vi "Call Steps.vi"(8 "error in (no error)":errorcluster, 11 "Cluster":T1={"Tite"="", "Base path"=path "", "Table"=[], "Stations"=[], "Shield Array"=[], "UPHs"=[], "VISA"={"VISA"="", "baud rate"=9600, "data bits"=8, "parity"=enum."None", "stop bits"=10, "flow control"=0}, "Path"={"roof"=path "", "Config"=path "", "Png"=path ""}, "Ctr"={"DB Dispaly"=refnum, "Error Table"=refnum, "Display"=refnum, "Login"=refnum, "Exit"=refnum, "FTT_Submit"=refnum}, "Login"={"User"="", "Grade"=""}, "information"={"cause"="", "Type"=enum."Inform", "code"=0, "Suroce"="", "Status"=FALSE}, "Local DB"={"Connstr"="", "Database"={"Constr"={"Driver"="", "Server"="", "User"="", "Pwd"="", "Database"=""}, "conn ref"=refnum, "State"=FALSE}}, "Remote DB"={"Connstr"="", "Database"={"Constr"={"Driver"="", "Server"="", "User"="", "Pwd"="", "Database"=""}, "conn ref"=refnum, "State"=FALSE}}, "FTT TV"="", "ExchangeTime"=0, "NVH"="", "EOL Path"=path ""} {"VISA"."flow control" items=["None", "XON/XOFF", "RTS/CTS", "XON/XOFF & RTS/CTS", "DTR/DSR", "XON/XOFF & DTR/DSR"]; "VISA"."stop bits" items=["1.0"=10, "1.5"=15, "2.0"=20]}) -> (0 "error out":errorcluster)   [LabVIEW 2014]
uses:
  Type'def/UPH Config.ctl
  VISA/Ctr/VISA Ctr.ctl
  Type'def/Main Ctr Ref.ctl
  Type'def/User Login.ctl
  Database/Ctr/Constr.ctl
  <vilib>/addons/database/Connection.llb/Conn ObjectReference.ctl
  <vilib>/addons/database/NI_Database_API.lvlib
  Database/Ctr/Conneect State.ctl
  Type'def/MainCtr.ctl
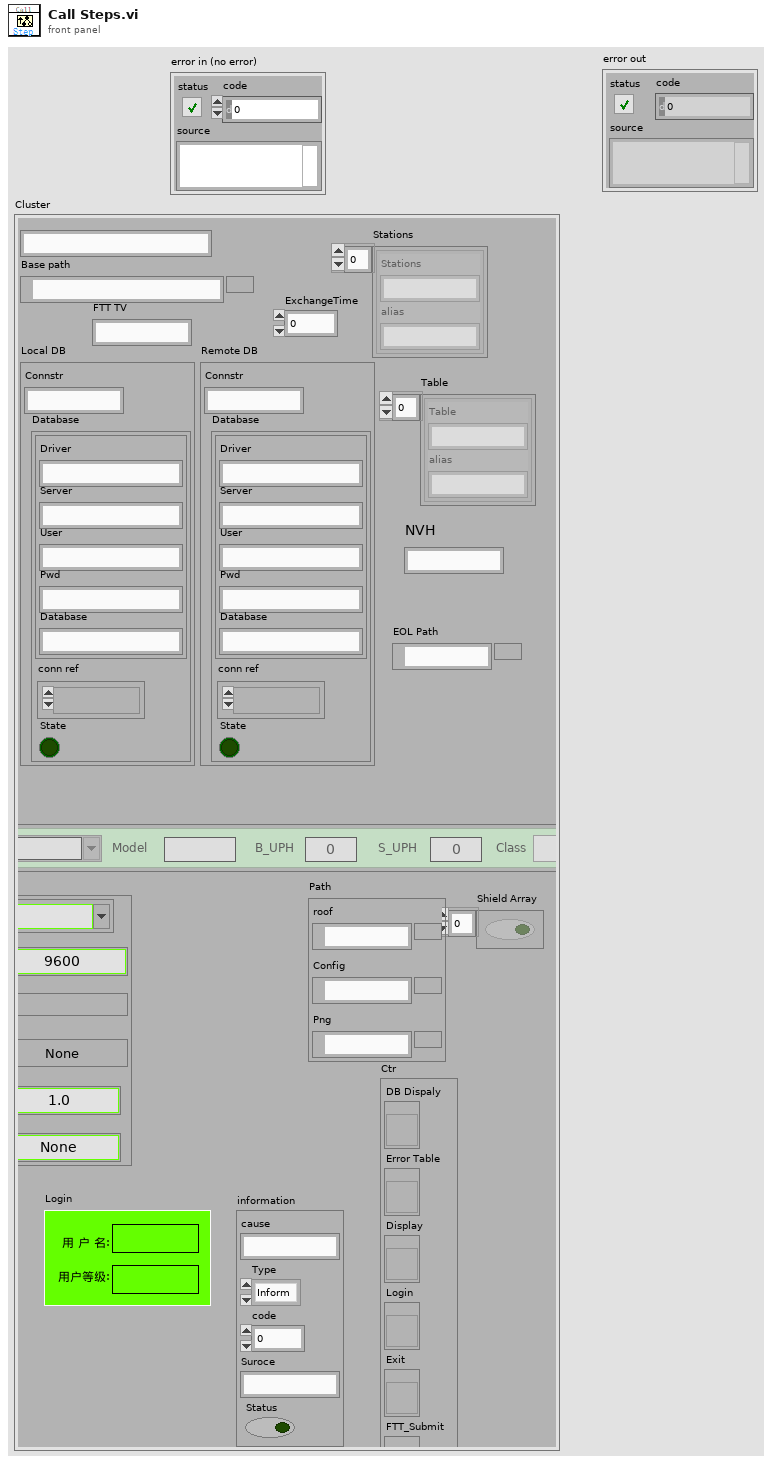
[diagram p1: front panel]
types:
  T1 = typedef "MainCtr.ctl" = cluster{"Tite":string, "Base path":path, "Table":cluster{"Table":string, "alias":string}[], "Stations":cluster{"Stations":string, "alias":string}[], "Shield Array":bool[], "UPHs":T2[], "VISA":T3, "Path":cluster{"roof":path, "Config":path, "Png":path}, "Ctr":T4, "Login":T5, "information":cluster{"cause":string, "Type":enum16{"Inform", "Warning", "Alarm"}, "code":i32, "Suroce":string, "Status":bool}, "Local DB":cluster{"Connstr":string, "Database":T6}, "Remote DB":cluster{"Connstr":string, "Database":T6}, "FTT TV":string, "ExchangeTime":i32, "NVH":string, "EOL Path":path}
  T2 = typedef "UPH Config.ctl" = cluster{"Line_No":string, "Model":string, "B_UPH ":i16, "S_UPH  ":i16, "Class":enum16{"Big", "Small"}}
  T3 = typedef "VISA Ctr.ctl" = cluster{"VISA":refnum<visa-resource-name>, "baud rate":u32, "data bits":u16, "parity":enum16{"None", "Odd", "Even", "Mark", "Space"}, "stop bits":u16, "flow control":u16}
  T4 = typedef "Main Ctr Ref.ctl" = cluster{"DB Dispaly":refnum<vi>, "Error Table":refnum<vi>, "Display":refnum<vi>, "Login":refnum<vi>, "Exit":refnum<vi>, "FTT_Submit":refnum<vi>}
  T5 = typedef "User Login.ctl" = cluster{"User":string, "Grade":string}
  T6 = typedef "Conneect State.ctl" = cluster{"Constr":T7, "conn ref":T8, "State":bool}
  T7 = typedef "Constr.ctl" = cluster{"Driver":string, "Server":string, "User":string, "Pwd":string, "Database":string}
  T8 = typedef "NI_Database_API.lvlib/Conn ObjectReference.ctl" = refnum<k1>
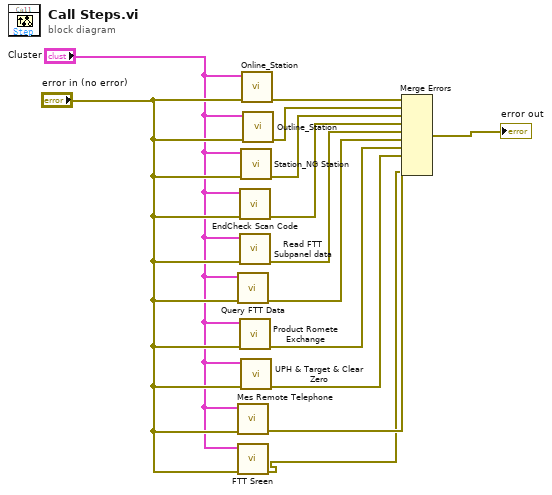
[diagram p0: block diagram]
diagram:
  n1 = call "Query FTT Data.vi"("error in (no error)"="error in (no error)", "Main"="Cluster") -> ("error out"=w7:errorcluster)  [unwired: 9 in]
  n2 = call "Mes Remote Telephone.vi"("error in (no error)"="error in (no error)", "Main"="Cluster") -> ("error out"=w4:errorcluster)  [unwired: 9 in]
  n3 = call "FTT Sreen.vi"("error in (no error)"="error in (no error)", "Main"="Cluster") -> ("error out"=w1:errorcluster)  [unwired: 9 in]
  n4 = call "EndCheck Scan Code.vi"("error in (no error)"="error in (no error)", "Main"="Cluster") -> ("error out"=w9:errorcluster)  [unwired: 9 in]
  n5 = call "Read FTT Subpanel data.vi"("error in (no error)"="error in (no error)", "Main"="Cluster") -> ("error out"=w8:errorcluster)  [unwired: 9 in]
  n6 = call "Product Romete Exchange.vi"("error in (no error)"="error in (no error)", "Main"="Cluster") -> ("error out"=w6:errorcluster)  [unwired: 9 in]
  n7 = call "Station_NG Station.vi"("error in (no error)"="error in (no error)", "Main"="Cluster") -> ("error out"=w10:errorcluster)  [unwired: 9 in]
  n8 = call "UPH & Target & Clear Zero.vi"("error in (no error)"="error in (no error)", "Main"="Cluster") -> ("error out"=w5:errorcluster)  [unwired: 9 in]
  n9 = call "Online_Station.vi"("error in (no error)"="error in (no error)", "Main"="Cluster") -> ("error out"=w13:errorcluster)  [unwired: 9 in]
  n10 = call "Outline_Station.vi"("error in (no error)"="error in (no error)", "Main"="Cluster") -> ("error out"=w12:errorcluster)  [unwired: 9 in]
  n11 = Merge Errors(w13, w12, w10, w9, w8, w7, w6, w5, w4, w1) -> (→"error out":errorcluster)
